vi "Taiko_Demo.vi"() -> ()   [LabVIEW 2010]
uses:
  Types/Taiko_Cmds.ctl
  Types/Taiko_Data.ctl
  _lib/PDLM/pdlm_lib_x86_x64_UIThread.llb/PDLM_Tag.ctl
  _lib/PDLM/pdlm_lib_x86_x64_UIThread.llb/PDLM_TaggedValue.ctl
  _lib/PDLM/pdlm_lib_x86_x64_UIThread.llb/PDLM_TaggedValueList.ctl
  <vilib>/Utility/miscctls.llb/LVRowAndColumnTypeDef.ctl
  _lib/PDLM/pdlm_lib_x86_x64_UIThread.llb/PDLM_TriggerMode.ctl
  Types/ControlAttributes.ctl
  Types/ScaleDisplayParams.ctl
  SubVIs/AddControlsToControlStateArray.vi
  _lib/PDLM/pdlm_lib_x86_x64_UIThread.llb/PDLM_PulseTableIDs.ctl
  Types/selector.ctl
panel:
  out "Info":string="Library Version:\n1.0.64.3114\n\nSerials:\n1234567\r\n"
  in  "SetSelector":T1 caption="Select:"
  in  "LDH Pulse Table IDs":T2
  in  "Slide":sgl(slide) min=0 max=100 step=0.1 scale=0.0..100.0
  out "Tagged Value List":i32[](listbox)
  out "SystemStatus":i32(listbox)=-1
  out "SystemStatusText":string="queued error message pending\nlocked by key lock\nlocked by on/off button\nparameter changes pending\nexclusive software operation granted"
  out "QError":string="queued error message pending\nlocked by key lock\nlocked by on/off button\nparameter changes pending\nexclusive software operation granted"
  out "LH Info & Data":i32(listbox)=-1
  out "LHFeatures":i32(listbox)=-1
  out "LHFeaturesText":string="pulse mode option (int. & ext. triggerable)\ncontinuous-wave option\nburst mode option (int. triggerable)\nfan-cooled (switchable)\nintensity sensor option (type=1)"
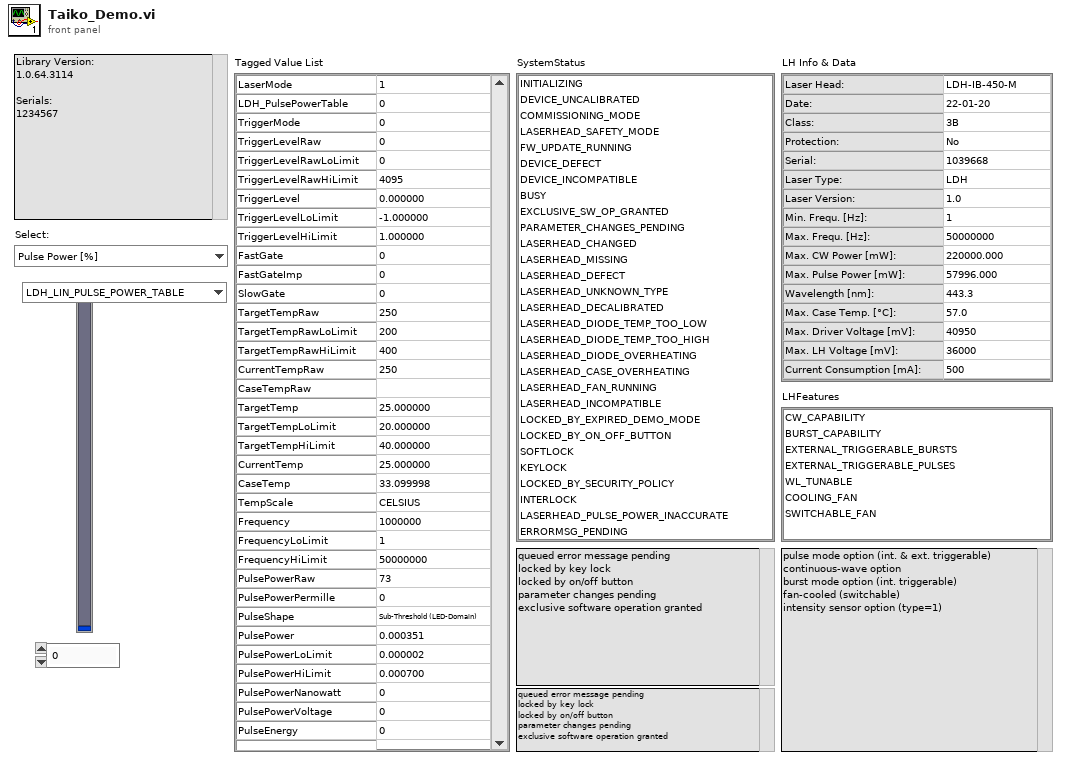
[diagram p1: front panel]
types:
  T1 = typedef "selector.ctl" = enum16{"Pulse Power [%]", "Frequency [Hz]", "Trigger Level [V]", "Pulse Table"}
  T2 = typedef "PDLM_PulseTableIDs.ctl" = enum16{"LDH_LIN_PULSE_POWER_TABLE", "LDH_MAX_PULSE_POWER_TABLE"}
  T3 = typedef "Taiko_Data.ctl" = cluster{"USBIdx":i32, "Error":errorcluster, "TaggedValueList":T4, "Ctrl State Arr":T7[], "Scale Display Params":T8}
  T4 = typedef "PDLM_TaggedValueList.ctl" = T5[]
  T5 = typedef "PDLM_TaggedValue.ctl" = cluster{"Tag":T6, "Value":u32}
  T6 = typedef "PDLM_Tag.ctl" = u32
  T7 = typedef "ControlAttributes.ctl" = cluster{"Ctl Refnum":refnum<vi>, "Visible":bool, "Enabled state":enum8{"Enabled", "Disabled", "Disabled and Grayed Out"}}
  T8 = typedef "ScaleDisplayParams.ctl" = cluster{"Style":u8, "MapMode":u8, "Increment":dbl, "Minimum":dbl, "Maximum":dbl, "Value":dbl}
  T9 = typedef "Taiko_Cmds.ctl" = enum16{"Idle", "Init", "Exit", "Update", "Error"}
  T10 = typedef "PDLM_TriggerMode.ctl" = enum32{"INTERNAL", "EXTERNAL_FALLING_EDGE", "EXTERNAL_RISING_EDGE"}
  T11 = typedef "LVRowAndColumnTypeDef.ctl" = cluster{"Row":i32, "Column":i32}
  T12 = enum16{"Pulse Power [%]", "Frequency [Hz]", "Trigger Level [V]"}
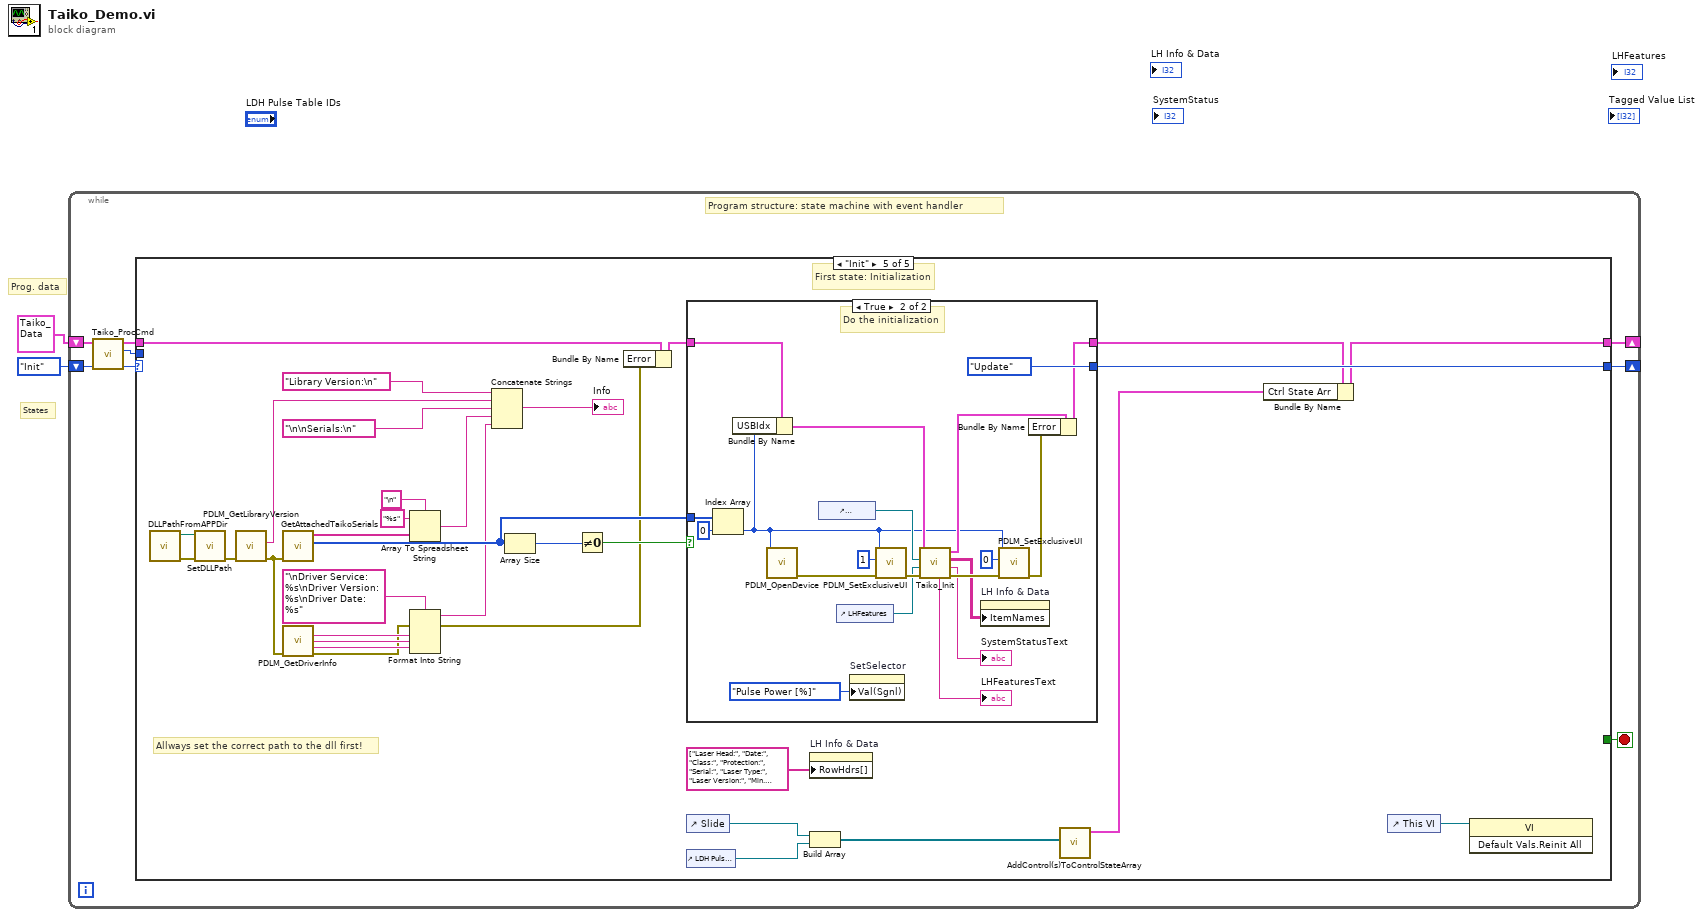
[diagram p0: block diagram]
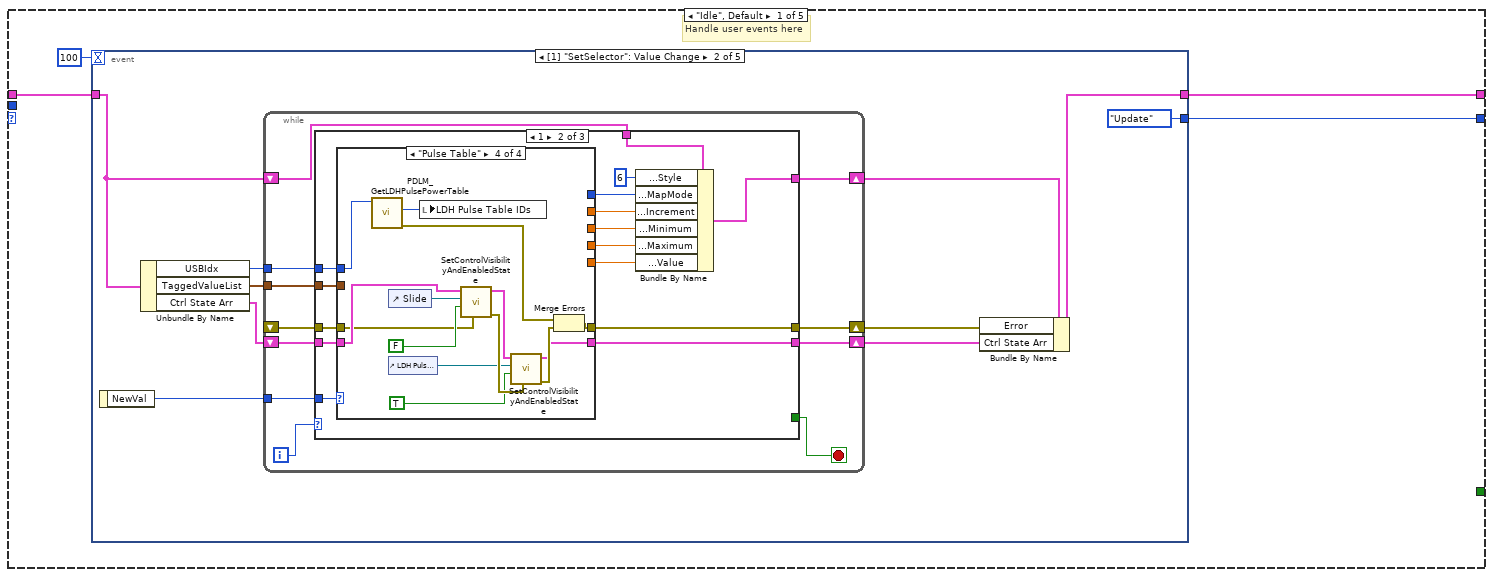
[diagram p2: hidden frame]
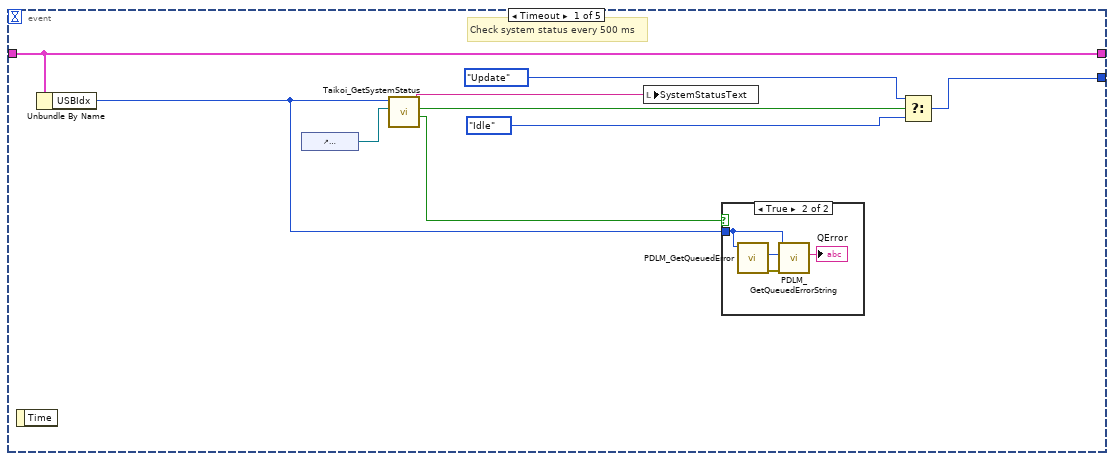
[diagram p3: hidden frame]
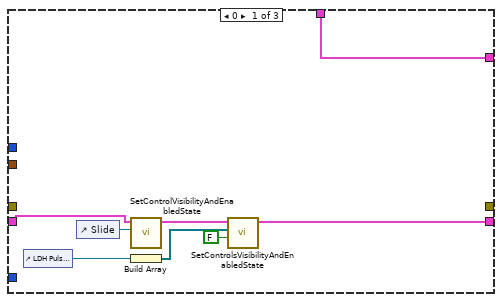
[diagram p5: hidden frame]
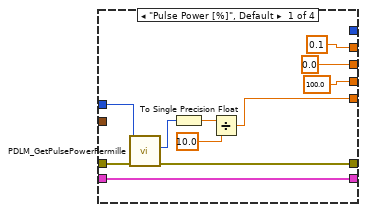
[diagram p6: hidden frame]
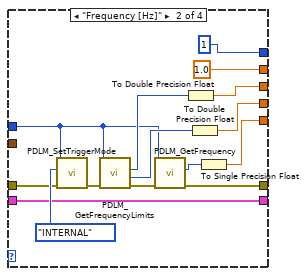
[diagram p7: hidden frame]
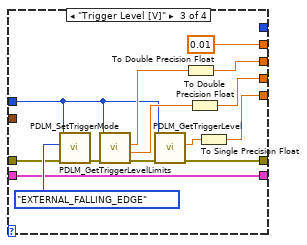
[diagram p8: hidden frame]
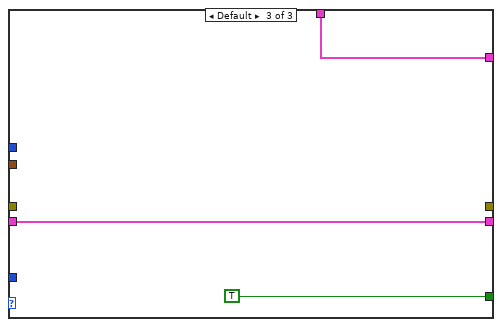
[diagram p9: hidden frame]
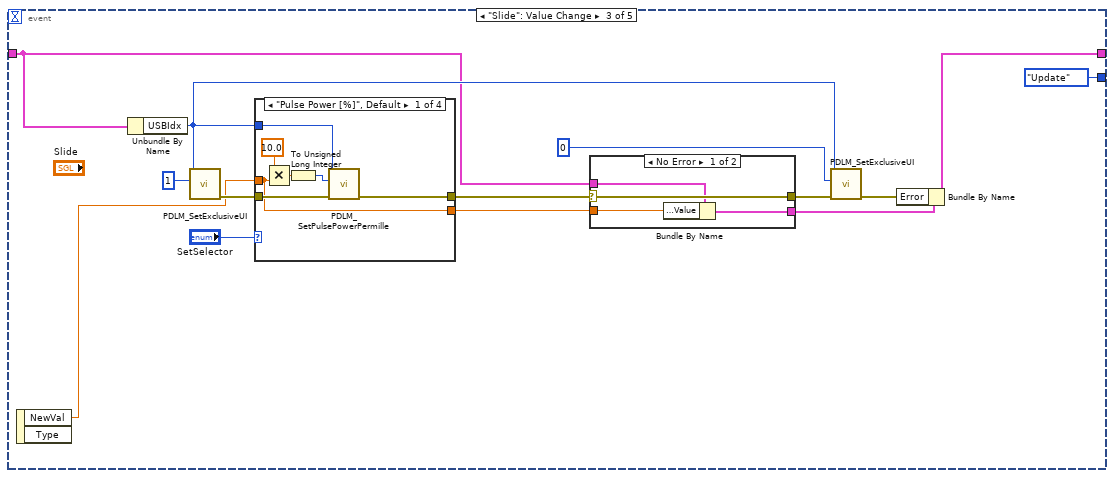
[diagram p10: hidden frame]
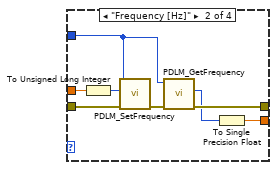
[diagram p12: hidden frame]
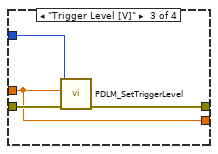
[diagram p13: hidden frame]
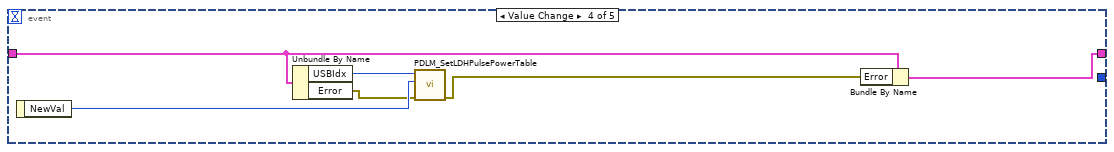
[diagram p15: hidden frame]
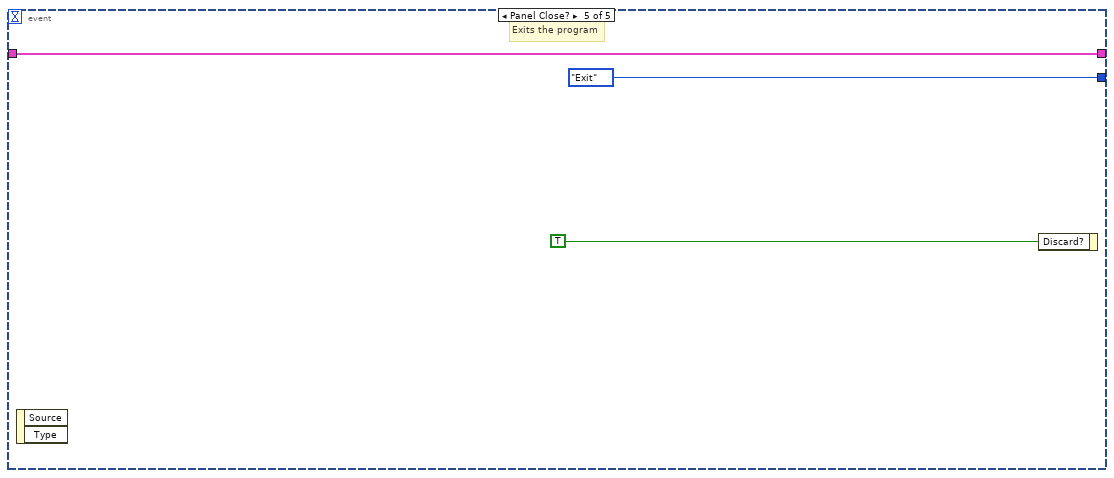
[diagram p16: hidden frame]
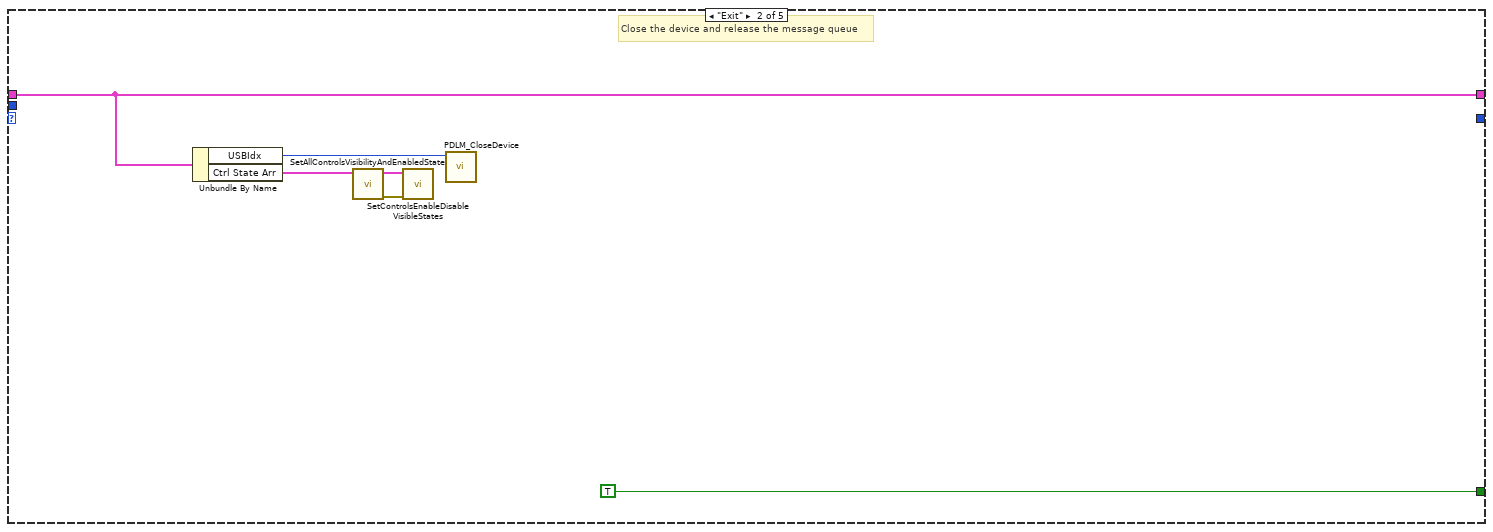
[diagram p17: hidden frame]
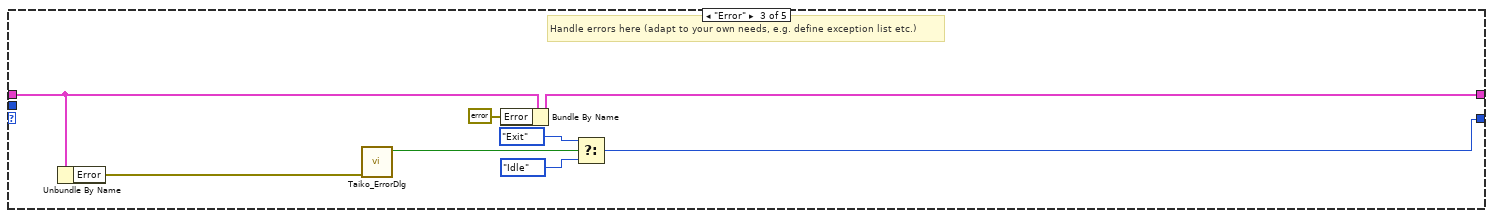
[diagram p18: hidden frame]
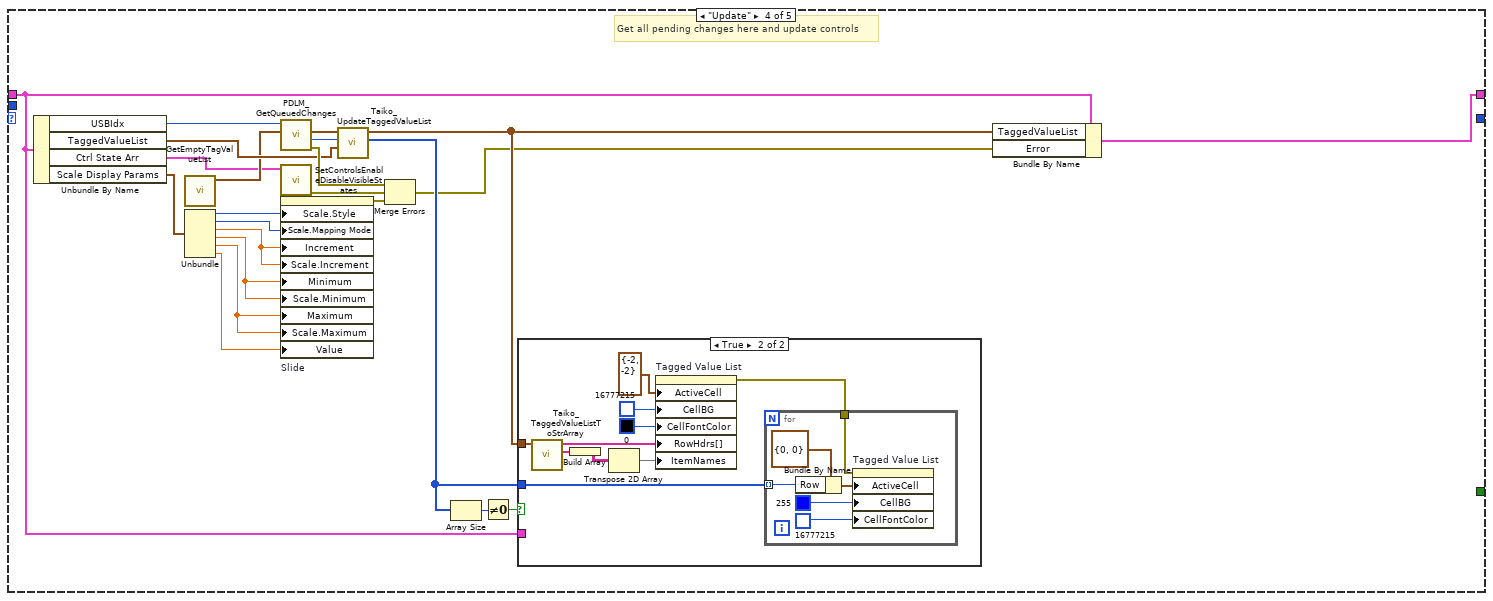
[diagram p19: hidden frame]
diagram:
  # "Prog. data"
  # "States"
  n1 = while {
    shift-right: [w9] -> _
    shift-left: Taiko_Cmds."Init" ("Cmd") -> [w5]
    shift-right: [w8] -> _
    shift-left: T3 {"USBIdx"=0, "Error"={"status"=FALSE, "code"=0, "source"=""}, "TaggedValueList"=[], "Ctrl State Arr"=[], "Scale Display Params"={"Style"=0, "MapMode"=0, "Increment"=0.0, "Minimum"=0.0, "Maximum"=0.0, "Value"=0.0}} ("Data") -> [w7]
    stop <- w10 stop-if-true
    # "Program structure: state machine with event handler"
    n2 = call "Taiko_ProcCmd.vi"("Cmd in"=w5, "Data in"=w7) -> ("Cmd out"=w4:T9, "Cmd prev"=w3:T9, "Data out"=w6:T3)  [unwired: 7 in]
    n3 = case shown="\"Init\"" w4 {
      tunnel: [_ TRUE _ _ _] -> w10
      tunnel: [w11 _ w187 _ w260] -> w9
      tunnel: w6 -> [w12 w183 w191 w206 w259]
      tunnel: [w13 w183 w190 w214 w244] -> w8
      tunnel: w3 -> [_ _ _ _ _]
      frame "Idle", Default {
        # "Handle user events here"
        n4 = event shown="[1] \"SetSelector\": Value Change" {
          selector: _ -> [_ _ _ _ _]
          dyn-events: _ -> [_ _ _ _ _]
          timeout: 100 -> [_ _ _ _ _]
          tunnel: [w19 Taiko_Cmds."Update" ("Cmd") Taiko_Cmds."Update" ("Cmd") _ Taiko_Cmds."Exit" ("Cmd")] -> w11
          tunnel: [w22 w35 w141 w171 w175] -> w13
          tunnel: w12 -> [w22 w29 w129 w172 w175]
          event Timeout {
            # "Check system status every 500 ms"
            n5 = event-data() -> ()  [unwired: 1 in, 1 out]
            n6 = Unbundle By Name(w22) -> ("USBIdx"=w15:i32)
            n7 = control-ref of="SystemStatus"() -> (w23:refnum<vi>)
            n8 = call "Taikoi_GetSystemStatus.vi"("LBSysStatRef"=w23, "USBIdx"=w15) -> ("QError"=w16:bool, "needUpdate"=w17:bool, "Status"=w18:string)  [unwired: 6 in, 1 out]
            n9 = local write "SystemStatusText"(w18) -> ()
            n10 = case shown="True" w16 {
              tunnel: w15 -> [_ w25]
              frame False {
              }
              frame True {
                n11 = call "PDLM_GetQueuedError.vi"("USBIdx"=w25) -> ("error out"=w27:errorcluster, "ErrCode"=w26:i32)  [unwired: 8 in, 1 out]
                n12 = call "PDLM_GetQueuedErrorString.vi"("error in (no error)"=w27, "ErrCode"=w26, "USBIdx"=w25) -> ("ErrText"=→"QError":string)  [unwired: 6 in, 2 out]
              }
            }
            n13 = Select(t=Taiko_Cmds."Update" ("Cmd"), s=w17, f=Taiko_Cmds."Idle") -> (s? t:f=w19:T9)
          }
          event Value Change {
            n14 = event-data() -> ("NewVal"=w36:T1)  [unwired: 1 in]
            n15 = Unbundle By Name(w29) -> ("USBIdx"=w37:i32, "TaggedValueList"=w33:T4, "Ctrl State Arr"=w31:T7[])
            n16 = while {
              tunnel: w37 -> [w48]
              tunnel: w36 -> [w47]
              tunnel: w33 -> [w45]
              shift-right: [w44] -> w32
              shift-left: w31 -> [w43]
              shift-right: [w46] -> w34
              shift-left: _ -> [w40]
              shift-right: [w38] -> w28
              shift-left: w29 -> [w39]
              i -> [w42]
              stop <- w41 stop-if-true
              n17 = case shown="1" w42 {
                tunnel: w48 -> [_ w71 _]
                tunnel: w47 -> [_ w70 _]
                tunnel: [_ w69 _] -> w46
                tunnel: w45 -> [_ w68 _]
                tunnel: [w50 w66 w127] -> w44
                tunnel: w43 -> [w52 w67 w127]
                tunnel: [_ _ TRUE] -> w41
                tunnel: w40 -> [_ w65 _]
                tunnel: w39 -> [w49 w64 w126]
                tunnel: [w49 w63 w126] -> w38
                frame 0 {
                  n18 = control-ref of="LDH Pulse Table IDs"() -> (w55:refnum<vi>)
                  n19 = control-ref of="Slide"() -> (w54:refnum<vi>)
                  n20 = call "SetControlVisibilityAndEnabledState.vi"("Ctl Refnum"=w54, "Control State Array"=w52) -> ("Control State Array (out)"=w53:T7[])  [unwired: 8 in, 1 out]
                  n21 = Build Array(w55) -> (w56:refnum<vi>[])
                  n22 = call "SetControlsVisibilityAndEnabledState.vi"("Visible (T)"=FALSE, "Array"=w56, "Control State Array"=w53) -> ("Control State Array (out)"=w50:T7[])  [unwired: 7 in, 1 out]
                }
                frame 1 {
                  n23 = case shown="\"Pulse Table\"" w70 {
                    tunnel: w71 -> [w79 w86 w101 w114]
                    tunnel: [0.0 w94 w109 _] -> w59
                    tunnel: [100.0 w92 w107 _] -> w58
                    tunnel: [w75 w90 w106 _] -> w57
                    tunnel: [w78 w96 w110 w113] -> w69
                    tunnel: [0.1 ("Data Entry Limits:Increment") 1.0 ("Data Entry Limits:Increment") 0.01 ("Data Entry Limits:Increment") _] -> w60
                    tunnel: [_ u8 1 ("Scale.Mapping Mode") _ _] -> w61
                    tunnel: w68 -> [_ _ _ _]
                    tunnel: w67 -> [w73 w84 w99 w122]
                    tunnel: [w73 w84 w99 w116] -> w66
                    tunnel: w65 -> [w72 w83 w98 w121]
                    frame "Pulse Power [%]", Default {
                      n24 = call "PDLM_GetPulsePowerPermille.vi"("error in (no error)"=w72, "USBIdx"=w79) -> ("error out"=w78:errorcluster, "permille"=w77:u32)  [unwired: 7 in, 1 out]
                      n25 = To Single Precision Float(number=w77) -> (single precision float=w76:sgl)
                      n26 = Divide(x=w76, y=sgl 10.0) -> (x/y=w75:sgl)
                    }
                    frame "Frequency [Hz]" {
                      n27 = call "PDLM_SetTriggerMode.vi"("error in (no error)"=w83, "mode"=PDLM_TriggerMode."INTERNAL", "USBIdx"=w86) -> ("error out"=w87:errorcluster)  [unwired: 7 in, 1 out]
                      n28 = call "PDLM_GetFrequencyLimits.vi"("error in (no error)"=w87, "USBIdx"=w86) -> ("error out"=w97:errorcluster, "MaxFreq"=w93:u32, "MinFreq"=w95:u32)  [unwired: 6 in, 1 out]
                      n29 = call "PDLM_GetFrequency.vi"("error in (no error)"=w97, "USBIdx"=w86) -> ("error out"=w96:errorcluster, "freq"=w91:u32)  [unwired: 7 in, 1 out]
                      n30 = To Double Precision Float(number=w95) -> (double precision float=w94:dbl)
                      n31 = To Double Precision Float(number=w93) -> (double precision float=w92:dbl)
                      n32 = To Single Precision Float(number=w91) -> (single precision float=w90:sgl)
                    }
                    frame "Trigger Level [V]" {
                      n33 = call "PDLM_SetTriggerMode.vi"("error in (no error)"=w98, "mode"=PDLM_TriggerMode."EXTERNAL_FALLING_EDGE", "USBIdx"=w101) -> ("error out"=w102:errorcluster)  [unwired: 7 in, 1 out]
                      n34 = call "PDLM_GetTriggerLevelLimits.vi"("error in (no error)"=w102, "USBIdx"=w101) -> ("error out"=w111:errorcluster, "MaxLevel"=w108:sgl, "MinLevel"=w104:sgl)  [unwired: 6 in, 1 out]
                      n35 = call "PDLM_GetTriggerLevel.vi"("error in (no error)"=w111, "USBIdx"=w101) -> ("error out"=w110:errorcluster, "Level"=w103:sgl)  [unwired: 7 in, 1 out]
                      n36 = To Double Precision Float(number=w104) -> (double precision float=w109:dbl)
                      n37 = To Double Precision Float(number=w108) -> (double precision float=w107:dbl)
                      n38 = To Single Precision Float(number=w103) -> (single precision float=w106:sgl)
                    }
                    frame "Pulse Table" {
                      n39 = call "PDLM_GetLDHPulsePowerTable.vi"("USBIdx"=w114) -> ("error out"=w112:errorcluster, "TableIdx (out)"=w115:u32)  [unwired: 8 in, 1 out]
                      n40 = control-ref of="Slide"() -> (w125:refnum<vi>)
                      n41 = control-ref of="LDH Pulse Table IDs"() -> (w118:refnum<vi>)
                      n42 = local write "LDH Pulse Table IDs"(w115) -> ()
                      n43 = call "SetControlVisibilityAndEnabledState.vi"("error in (no error)"=w121, "Visible (T)"=FALSE, "Ctl Refnum"=w125, "Control State Array"=w122) -> ("error out"=w120:errorcluster, "Control State Array (out)"=w124:T7[])  [unwired: 6 in]
                      n44 = call "SetControlVisibilityAndEnabledState.vi"("error in (no error)"=w120, "Visible (T)"=TRUE, "Ctl Refnum"=w118, "Control State Array"=w124) -> ("error out"=w119:errorcluster, "Control State Array (out)"=w116:T7[])  [unwired: 6 in]
                      n45 = Merge Errors(w112, w119) -> (w113:errorcluster)
                    }
                  }
                  n46 = Bundle By Name(cluster=w64, "Scale Display Params.Style"=u8 6, "Scale Display Params.MapMode"=w61, "Scale Display Params.Increment"=w60, "Scale Display Params.Minimum"=w59, "Scale Display Params.Maximum"=w58, "Scale Display Params.Value"=w57) -> (w63:T3)
                }
                frame Default {
                }
              }
            }
            n47 = Bundle By Name(cluster=w28, "Error"=w34, "Ctrl State Arr"=w32) -> (w35:T3)
          }
          event "Slide": Value Change {
            n48 = event-data() -> ("NewVal"=w131:sgl)  [unwired: 1 in, 1 out]
            n49 = Unbundle By Name(w129) -> ("USBIdx"=w137:i32)
            n50 = call "PDLM_SetExclusiveUI.vi"("mode"=u32 1, "USBIdx"=w137) -> ("error out"=w140:errorcluster)  [unwired: 8 in, 1 out]
            n51 = case shown="\"Pulse Power [%]\", Default" "SetSelector" {
              tunnel: w137 -> [w155 w157 w167 _]
              tunnel: w131 -> [w149 w158 w164 _]
              tunnel: [w151 w162 w165 w168] -> w134
              tunnel: w140 -> [w154 w163 w166 w168]
              tunnel: [w149 w156 w164 _] -> w130
              frame "Pulse Power [%]", Default {
                n52 = Multiply(x=sgl 10.0, y=w149) -> (x*y=w152:sgl)
                n53 = To Unsigned Long Integer(number=w152) -> (unsigned 32bit integer=w150:u32)
                n54 = call "PDLM_SetPulsePowerPermille.vi"("error in (no error)"=w154, "permille"=w150, "USBIdx"=w155) -> ("error out"=w151:errorcluster)  [unwired: 7 in, 1 out]
              }
              frame "Frequency [Hz]" {
                n55 = To Unsigned Long Integer(number=w158) -> (unsigned 32bit integer=w160:u32)
                n56 = call "PDLM_SetFrequency.vi"("error in (no error)"=w163, "freq"=w160, "USBIdx"=w157) -> ("error out"=w161:errorcluster)  [unwired: 7 in, 1 out]
                n57 = call "PDLM_GetFrequency.vi"("error in (no error)"=w161, "USBIdx"=w157) -> ("error out"=w162:errorcluster, "freq"=w159:u32)  [unwired: 7 in, 1 out]
                n58 = To Single Precision Float(number=w159) -> (single precision float=w156:sgl)
              }
              frame "Trigger Level [V]" {
                n59 = call "PDLM_SetTriggerLevel.vi"("error in (no error)"=w166, "Level"=w164, "USBIdx"=w167) -> ("error out"=w165:errorcluster)  [unwired: 7 in, 1 out]
              }
              frame "Pulse Table" {
              }
            }
            n60 = case shown="No Error" w134 {
              selector: w134 -> [w146 w147]
              tunnel: [w146 w147] -> w133
              tunnel: w129 -> [w145 w148]
              tunnel: [w144 w148] -> w132
              tunnel: w130 -> [w143 _]
              frame No Error {
                n61 = Bundle By Name(cluster=w145, "Scale Display Params.Value"=w143) -> (w144:T3)
              }
              frame Error {
              }
            }
            n62 = call "PDLM_SetExclusiveUI.vi"("error in (no error)"=w133, "mode"=u32 0, "USBIdx"=w137) -> ("error out"=w138:errorcluster)  [unwired: 7 in, 1 out]
            n63 = Bundle By Name(cluster=w132, "Error"=w138) -> (w141:T3)
          }
          event Value Change {
            n64 = event-data() -> ("NewVal"=w170:T2)  [unwired: 1 in]
            n65 = Unbundle By Name(w172) -> ("USBIdx"=w174:i32, "Error"=w169:errorcluster)
            n66 = call "PDLM_SetLDHPulsePowerTable.vi"("error in (no error)"=w169, "TableIdx"=w170, "USBIdx"=w174) -> ("error out"=w173:errorcluster)  [unwired: 7 in, 1 out]
            n67 = Bundle By Name(cluster=w172, "Error"=w173) -> (w171:T3)
          }
          event Panel Close? {
            # "Exits the program"
            n68 = event-data() -> ()  [unwired: 1 in, 2 out]
            n69 = event-data("Discard?"=TRUE) -> ()  [unwired: 1 in, 1 out]
          }
        }
      }
      frame "Exit" {
        # "Close the device and release the message queue"
        n70 = Unbundle By Name(w183) -> ("USBIdx"=w182:i32, "Ctrl State Arr"=w180:T7[])
        n71 = call "SetAllControlsVisibilityAndEnabledState.vi"("Control State Array"=w180) -> ("error out"=w178:errorcluster, "Control State Array (out)"=w179:T7[])  [unwired: 9 in]
        n72 = call "SetControlsEnableDisableVisibleStates.vi"("error in (no error)"=w178, "Array"=w179) -> ()  [unwired: 9 in, 1 out]
        n73 = call "PDLM_CloseDevice.vi"("USBIdx"=w182) -> ()  [unwired: 9 in, 2 out]
      }
      frame "Error" {
        # "Handle errors here (adapt to your own needs, e.g. define exception list etc.)"
        n74 = Unbundle By Name(w191) -> ("Error"=w185:errorcluster)
        n75 = call "Taiko_ErrorDlg.vi"("Error in"=w185) -> ("Exit"=w189:bool)  [unwired: 9 in, 1 out]
        n76 = Bundle By Name(cluster=w191, "Error"=errorcluster {"status"=FALSE, "code"=0, "source"=""}) -> (w190:T3)
        n77 = Select(t=Taiko_Cmds."Exit" ("Cmd"), s=w189, f=Taiko_Cmds."Idle") -> (s? t:f=w187:T9)
      }
      frame "Update" {
        # "Get all pending changes here and update controls"
        n78 = Unbundle By Name(w206) -> ("USBIdx"=w205:i32, "TaggedValueList"=w204:T4, "Ctrl State Arr"=w202:T7[], "Scale Display Params"=w200:T8)
        n79 = call "GetEmptyTagValueList.vi"() -> ("Array"=w203:T5[])  [unwired: 10 in, 1 out]
        n80 = Unbundle(w200) -> ("Style"=w199:u8, "MapMode"=w198:u8, "Increment"=w197:dbl, "Minimum"=w196:dbl, "Maximum"=w195:dbl, "Value"=w194:dbl)
        n81 = call "PDLM_GetQueuedChanges.vi"("TaggedValueList"=w203, "USBIdx"=w205) -> ("error out"=w213:errorcluster, "ListLen out"=w212:u32, "TaggedValueList out"=w211:T4)  [unwired: 6 in, 1 out]
        n82 = call "SetControlsEnableDisableVisibleStates.vi"("Array"=w202) -> ("error out"=w201:errorcluster)  [unwired: 10 in]
        n83 = property on="Slide" class="Slide (strict)"("Scale.Style"=w199, "Scale.Mapping Mode"=w198, "Increment"=w197, "Scale.Increment"=w197, "Minimum"=w196, "Scale.Minimum"=w196, "Maximum"=w195, "Scale.Maximum"=w195, "Value"=w194) -> (error out=w192:errorcluster)  [unwired: 2 in, 1 out]
        n84 = call "Taiko_UpdateTaggedValueList.vi"("TaggedValueList all"=w204, "ListLen in"=w212, "TaggedValueList in"=w211) -> ("Array"=w209:i32[], "TaggedValueList"=w210:T4)  [unwired: 7 in]
        n85 = Merge Errors(w213, w201, w192) -> (w193:errorcluster)
        n86 = Array Size(array=w209) -> (size(s)=w208:i32)
        n87 = Not Equal To 0?(x=w208) -> (x != 0?=w207:bool)
        n88 = case shown="True" w207 {
          tunnel: w210 -> [_ w220]
          tunnel: w209 -> [_ w215]
          tunnel: w206 -> [_ _]
          frame False {
          }
          frame True {
            n89 = call "Taiko_TaggedValueListToStrArray.vi"("TaggedValueList"=w220) -> ("ValList"=w221:string[], "TagList"=w223:string[])  [unwired: 9 in]
            n90 = Build Array(w221) -> (w222:string[][])
            n91 = Transpose 2D Array(2D array=w222) -> (transposed array=w224:string[][])
            n92 = property on="Tagged Value List" class="MCListbox (strict)"("ActiveCell"=T11 {"Row"=-2, "Column"=-2} ("Active Cell:Active Cell"), "CellBG"=u32 16777215, "CellFontColor"=u32 0, "RowHdrs[]"=w223, "ItemNames"=w224) -> (error out=w216:errorcluster)  [unwired: 2 in, 1 out]
            n93 = for {
              tunnel: w215 -> [w229] mode=indexing
              tunnel: w216 -> [w225]
              n94 = Bundle By Name(cluster=T11 {"Row"=0, "Column"=0} ("Active Cell:Active Cell"), "Row"=w229) -> (w228:T11)
              n95 = property on="Tagged Value List" class="MCListbox (strict)"(error in=w225, "ActiveCell"=w228, "CellBG"=u32 255 ("Color Box"), "CellFontColor"=u32 16777215) -> ()  [unwired: 1 in, 2 out]
            }
          }
        }
        n96 = Bundle By Name(cluster=w206, "TaggedValueList"=w210, "Error"=w193) -> (w214:T3)
      }
      frame "Init" {
        # "Allways set the correct path to the dll first!"
        # "First state: Initialization"
        n97 = call "DLLPathFromAPPDir.vi"() -> ("error out"=w232:errorcluster, "DLLPath"=w248:path)  [unwired: 10 in]
        n98 = call "SetDLLPath.vi"("error in (no error)"=w232, "DLLPath"=w248) -> ("error out"=w231:errorcluster)  [unwired: 9 in]
        n99 = call "PDLM_GetLibraryVersion.vi"("error in (no error)"=w231) -> ("error out"=w233:errorcluster, "Version"=w255:string)  [unwired: 8 in, 1 out]
        n100 = call "GetAttachedTaikoSerials.vi"("error in (no error)"=w233) -> ("Array 2"=w261:i32[], "Array"=w253:string[])  [unwired: 9 in]
        n101 = call "PDLM_GetDriverInfo.vi"("error in (no error)"=w233) -> ("cName"=w240:string, "cVersion"=w239:string, "cDate"=w238:string, "error out"=w235:errorcluster)  [unwired: 10 in, 1 out]
        n102 = Array To Spreadsheet String(delimiter (Tab)="\n", array=w253, 3:"%s" ("format string")) -> (spreadsheet string=w254:string)
        n103 = Format Into String(format string="\nDriver Service: %s\nDriver Version: %s\nDriver Date: %s" ("string"), error in=w235, w240, w239, w238) -> (resulting string=w234:string, error out=w236:errorcluster)  [unwired: 1 in]
        n104 = Concatenate Strings("Library Version:\n" ("string"), w255, "\n\nSerials:\n" ("string"), w254, w234) -> (→"Info":string)
        n105 = Array Size(array=w261) -> (size(s)=w263:i32)
        n106 = Not Equal To 0?(x=w263) -> (x != 0?=w262:bool)
        n107 = Bundle By Name(cluster=w259, "Error"=w236) -> (w237:T3)
        n108 = case shown="True" w262 {
          tunnel: w261 -> [_ w284]
          tunnel: [Taiko_Cmds."Exit" ("Cmd") Taiko_Cmds."Update" ("Cmd")] -> w260
          tunnel: w237 -> [w264 w273]
          tunnel: [w264 w280] -> w258
          frame False {
            # "No device to open found"
          }
          frame True {
            # "Do the initialization"
            n109 = Index Array(array=w284, index=0) -> (element=w268:i32)
            n110 = Bundle By Name(cluster=w273, "USBIdx"=w268) -> (w272:T3)
            n111 = call "PDLM_OpenDevice.vi"("USBIdx"=w268) -> ("error out"=w266:errorcluster)  [unwired: 8 in, 2 out]
            n112 = control-ref of="SystemStatus"() -> (w275:refnum<vi>)
            n113 = control-ref of="LHFeatures"() -> (w274:refnum<vi>)
            n114 = property on="SetSelector" class="Enum (strict)"("Val(Sgnl)"=T12."Pulse Power [%]" ("Value (Signaling)")) -> ()  [unwired: 2 in, 2 out]
            n115 = call "PDLM_SetExclusiveUI.vi"("error in (no error)"=w266, "mode"=u32 1, "USBIdx"=w268) -> ("error out"=w278:errorcluster)  [unwired: 7 in, 1 out]
            n116 = call "Taiko_Init.vi"("error in (no error)"=w278, "LBLHFeaturesRef"=w274, "LBSysStatRef"=w275, "Data"=w272) -> ("error out"=w277:errorcluster, "Status"=→"SystemStatusText":string, "LHInfoData"=w271:string[][], "Data out"=w269:T3, "Features"=→"LHFeaturesText":string)  [unwired: 3 in]
            n117 = property on="LH Info & Data" class="MCListbox (strict)"("ItemNames"=w271) -> ()  [unwired: 2 in, 2 out]
            n118 = call "PDLM_SetExclusiveUI.vi"("error in (no error)"=w277, "mode"=u32 0, "USBIdx"=w268) -> ("error out"=w279:errorcluster)  [unwired: 7 in, 1 out]
            n119 = Bundle By Name(cluster=w269, "Error"=w279) -> (w280:T3)
          }
        }
        n120 = control-ref of="Slide"() -> (w247:refnum<vi>)
        n121 = control-ref of="LDH Pulse Table IDs"() -> (w246:refnum<vi>)
        n122 = property on="LH Info & Data" class="MCListbox (strict)"("RowHdrs[]"=string[] ["Laser Head:", "Date:", "Class:", "Protection:", "Serial:", "Laser Type:", "Laser Version:", "Min. Frequ. [Hz]:", "Max. Frequ. [Hz]:", "Max. CW Power [mW]:", "Max. Pulse Power [mW]:", "Wavelength [nm]:", "Max. Case Temp. [°C]:", "Max. Driver Voltage [mV]:", "Max. LH Voltage [mV]:", "Current Consumption [mA]:", "Calib. Warranty [h]:"] ("Row Header Strings[]")) -> ()  [unwired: 2 in, 2 out]
        n123 = Build Array(w247, w246) -> (w245:refnum<vi>[])
        n124 = call-poly "AddControl(s)ToControlStateArray.vi"("Array"=w245) -> ("Control State Array (out)"=w243:T7[])  [unwired: 9 in, 1 out]
        n125 = Bundle By Name(cluster=w258, "Ctrl State Arr"=w243) -> (w244:T3)
        n126 = control-ref of="This VI"() -> (w242:refnum<vi>)
        n127 = invoke class="VI" method="Default Vals.Reinit All"(reference=w242) -> ()  [unwired: 2 in, 3 out]
      }
    }
  }
